vi "CRYOpen Curve Excel .vi"(11 "file path (dialog if empty)":path=path "D:/3_Doc/KTH/test excel/CRY6151 Data Col.csv") -> (0 "Return":bool, 3 "Data":T1[](array[typedef]) {"Z data" items=["dB", "Lin"]; "X data" items=["dB", "Lin"]; "Y data" items=["dB", "Lin"]; "Z dB ref" format="%.1f"; "Z axis" items=["Log", "Lin"]; "X dB ref" format="%.1f"; "X axis" items=["Log", "Lin"]; "Y axis" items=["Log", "Lin"]; "Y dB ref" format="%.1f"; "Curve"."z" format="%.2f"; "Curve"."y" format="%.2f"; "Curve"."x" format="%.2f"})   [LabVIEW 2013]
uses:
  Typedef Control/CRYData Cluster.ctl
  <vilib>/Utility/file.llb/Read From Spreadsheet File (string).vi
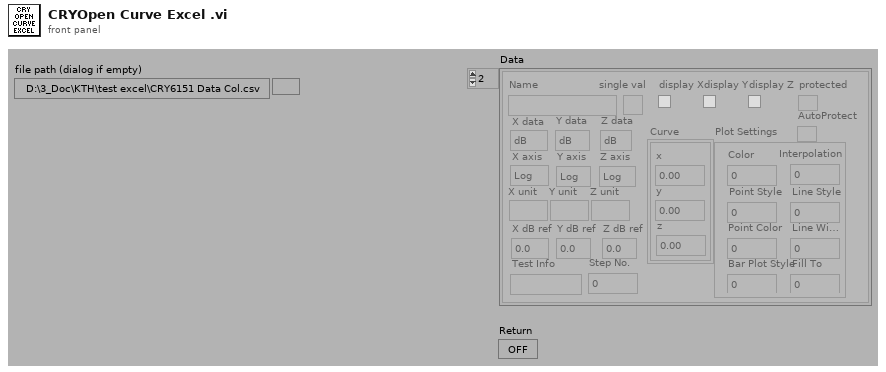
[diagram p1: front panel]
types:
  T1 = typedef "CRYData Cluster.ctl" = cluster{"Name":string, "Curve":cluster{"x":dbl, "y":dbl, "z":dbl}[], "X data":u16, "Y data":u16, "Z data":u16, "X axis":u16, "Y axis":u16, "Z axis":u16, "X unit":string, "Y unit":string, "Z unit":string, "X dB ref":dbl, "Y dB ref":dbl, "Z dB ref":dbl, "single val":bool, "protected":bool, "display X":bool, "display Y":bool, "display Z":bool, "Test Info":string, "Step No.":i32, "Plot Settings":cluster{"Color":u32, "Interpolation":u8, "Point Style":u8, "Line Style":u8, "Point Color":u32, "Line Width":u8, "Bar Plot Style":u8, "Fill To":i16}, "AutoProtect":bool}
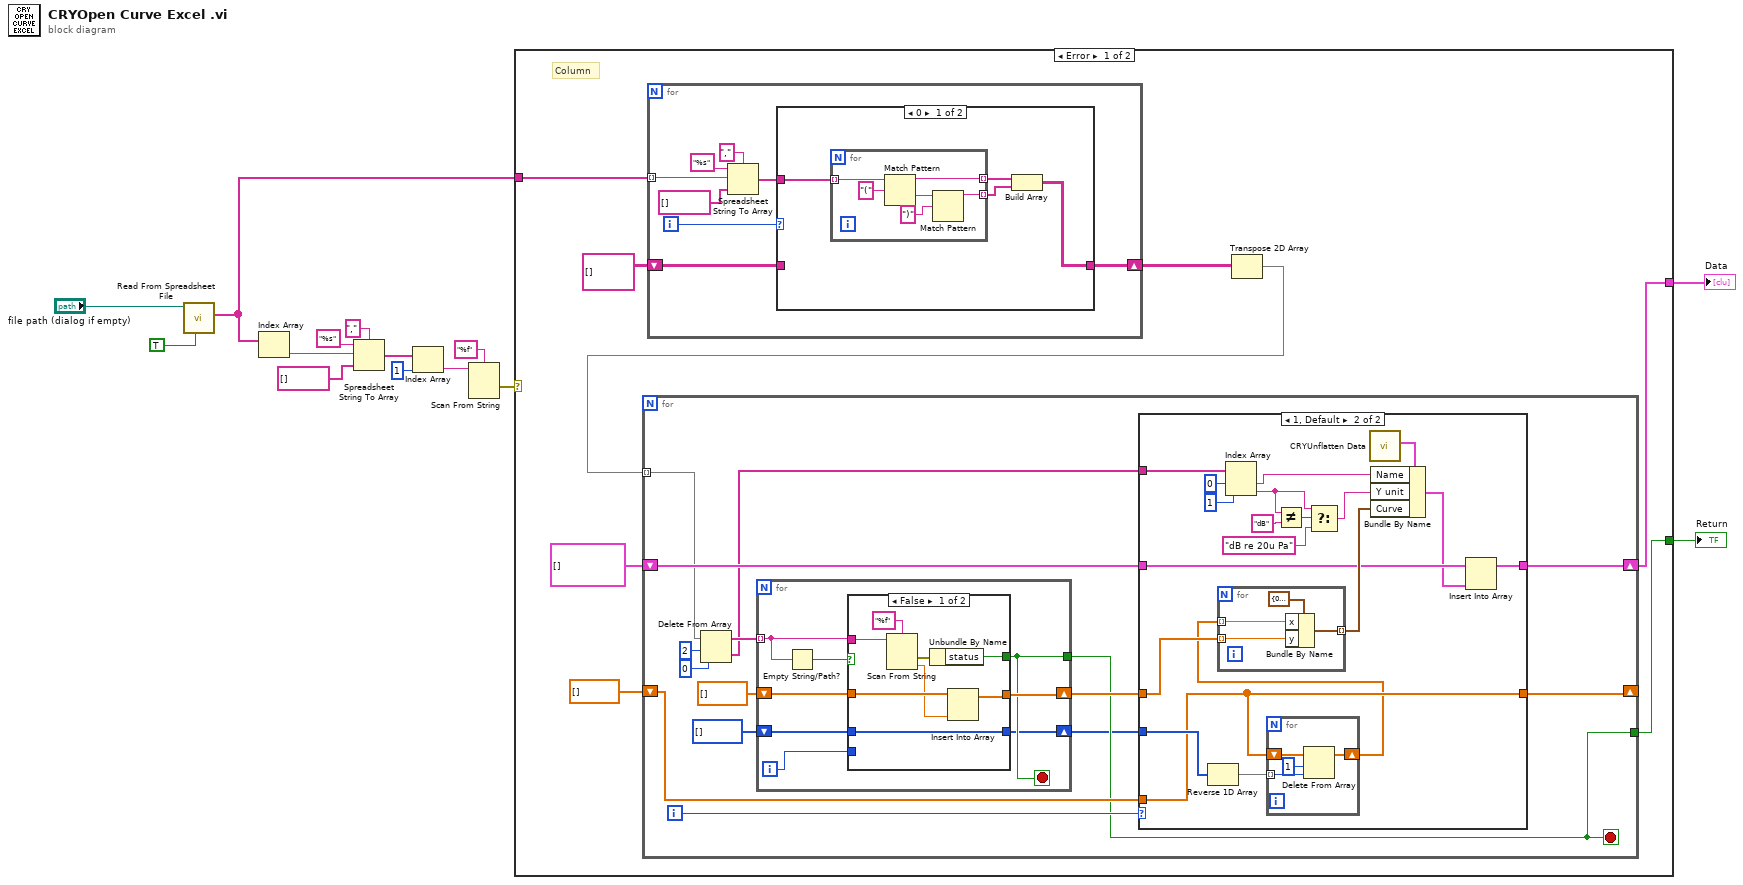
[diagram p0: block diagram]
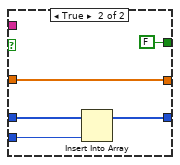
[diagram p3: hidden frame]
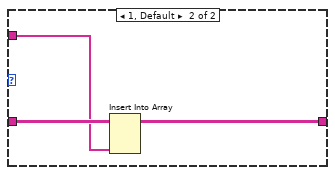
[diagram p4: hidden frame]
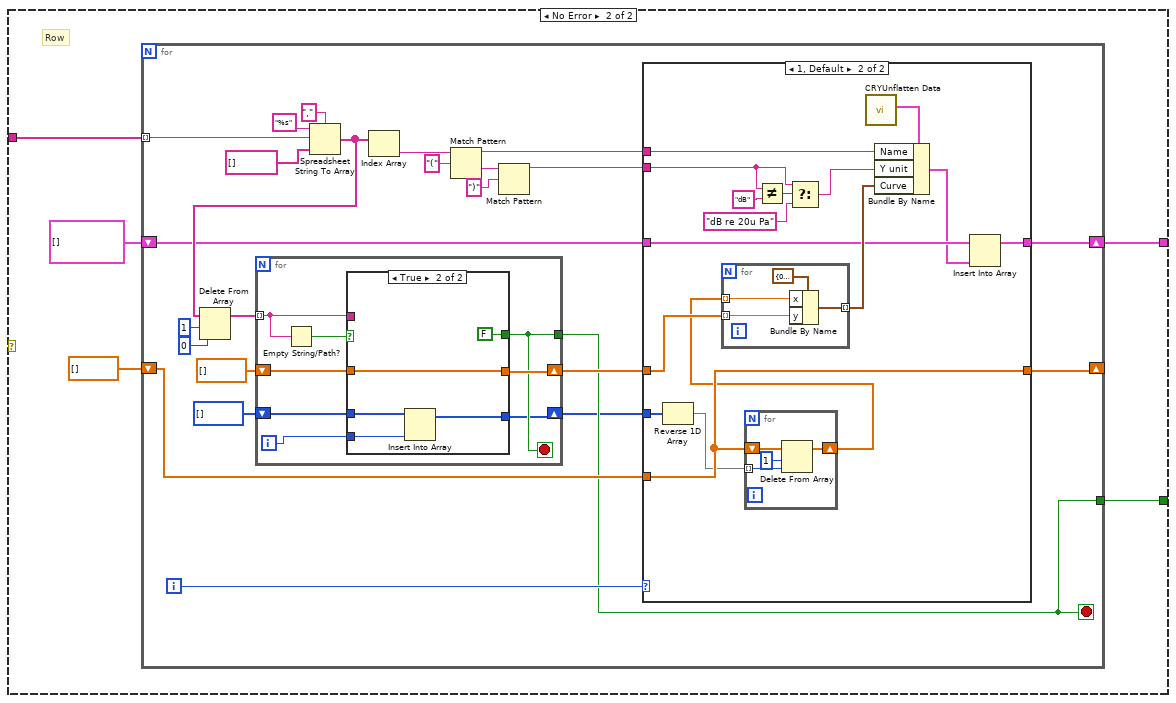
[diagram p5: hidden frame]
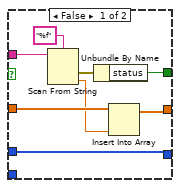
[diagram p7: hidden frame]
diagram:
  n1 = call-poly <vilib>:"Read From Spreadsheet File.vi"("transpose (no:F)"=TRUE, "file path (dialog if empty)"="file path (dialog if empty)") -> ("first row"=w3:string[])  [unwired: 5 in, 4 out]
  n2 = Index Array(array=w3) -> (element=w8:string)  [unwired: 1 in]
  n3 = Spreadsheet String To Array(delimiter (Tab)=",", format string="%s", spreadsheet string=w8, array type (2D Dbl)=string[] []) -> (array=w12:string[])
  n4 = Index Array(array=w12, index=1) -> (element=w5:string)
  n5 = Scan From String(format string="%f", input string=w5) -> (error out=w2:errorcluster)  [unwired: 4 in, 2 out]
  n6 = case shown="Error" w2 {
    tunnel: [w16 w111] -> w4
    tunnel: w3 -> [w22 w110]
    tunnel: [w15 w109] -> w1
    frame Error {
      # "Column"
      n7 = for {
        tunnel: w22 -> [w95] mode=indexing
        shift-right: [w88] -> w20
        shift-left: string[][] [] ("appended array") -> [w89]
        i -> [w90]
        n8 = Spreadsheet String To Array(delimiter (Tab)=",", format string="%s", spreadsheet string=w95, array type (2D Dbl)=string[] []) -> (array=w91:string[])
        n9 = case shown="0" w90 {
          tunnel: w91 -> [w99 w107]
          tunnel: [w97 w106] -> w88
          tunnel: w89 -> [_ w108]
          frame 0 {
            n10 = for {
              tunnel: w99 -> [w100] mode=indexing
              tunnel: [w102] -> w98 mode=indexing
              tunnel: [w101] -> w96 mode=indexing
              n11 = Match Pattern(string=w100, regular expression="(" ("search string/char (-)")) -> (before substring=w102:string, after substring=w105:string)  [unwired: 1 in, 2 out]
              n12 = Match Pattern(string=w105, regular expression=")") -> (before substring=w101:string)  [unwired: 1 in, 3 out]
            }
            n13 = Build Array(w98, w96) -> (w97:string[][])
          }
          frame 1, Default {
            n14 = Insert Into Array(array=w108, new element=w107) -> (w106:string[][])  [unwired: 2 in]
          }
        }
      }
      n15 = Transpose 2D Array(2D array=w20) -> (transposed array=w17:string[][])
      n16 = for {
        tunnel: w17 -> [w27] mode=indexing
        shift-right: [w31] -> _
        shift-left: dbl[] [] -> [w30]
        shift-right: [w28] -> w16
        shift-left: T1[] [] -> [w29]
        tunnel: [w25] -> w15
        i -> [w33]
        stop <- w25 stop-if-true
        n17 = Delete From Array(array=w27, length=2, index=0) -> (deleted portion=w26:string[], array with subset deleted=w35:string[])
        n18 = for {
          tunnel: w35 -> [w74] mode=indexing
          shift-right: [w71] -> w32
          shift-left: dbl[] [] -> [w72]
          tunnel: [w70] -> w25
          shift-right: [w68] -> w23
          shift-left: i32[] [] -> [w69]
          i -> [w67]
          stop <- w70 stop-if-true
          n19 = Empty String/Path?(string/path=w74) -> (empty?=w73:bool)
          n20 = case shown="False" w73 {
            tunnel: w74 -> [w81 _]
            tunnel: w72 -> [w80 w87]
            tunnel: [w79 w87] -> w71
            tunnel: [w76 FALSE ("status")] -> w70
            tunnel: w69 -> [w75 w85]
            tunnel: [w75 w84] -> w68
            tunnel: w67 -> [_ w83]
            frame False {
              n21 = Scan From String(format string="%f", input string=w81) -> (error out=w77:errorcluster, output 1=w78:dbl)  [unwired: 3 in, 2 out]
              n22 = Unbundle By Name(w77) -> ("status"=w76:bool)
              n23 = Insert Into Array(array=w80, new element=w78) -> (w79:dbl[])  [unwired: 1 in]
            }
            frame True {
              n24 = Insert Into Array(array=w85, new element=w83) -> (w84:i32[])  [unwired: 1 in]
            }
          }
        }
        n25 = case shown="1, Default" w33 {
          tunnel: w32 -> [w39 w56]
          tunnel: [w39 w46] -> w31
          tunnel: w30 -> [_ w46]
          tunnel: w29 -> [w38 w55]
          tunnel: [w38 w53] -> w28
          tunnel: w26 -> [_ w52]
          tunnel: w23 -> [_ w47]
          frame 0 {
          }
          frame 1, Default {
            n26 = Reverse 1D Array(array=w47) -> (reversed array=w48:i32[])
            n27 = Index Array(array=w52, index #1=0 ("index"), index #2=1 ("index")) -> (element #1=w49:string, element #2=w42:string)
            n28 = for {
              shift-right: [w59] -> w45
              shift-left: w46 -> [w62]
              tunnel: w48 -> [w61] mode=indexing
              n29 = Delete From Array(array=w62, length=1, index=w61) -> (array with subset deleted=w59:dbl[])  [unwired: 1 out]
            }
            n30 = for {
              tunnel: [w65] -> w57 mode=indexing
              tunnel: w45 -> [w64] mode=indexing
              tunnel: w56 -> [w63] mode=indexing
              n31 = Bundle By Name(cluster=cluster{"x":dbl, "y":dbl, "z":dbl} {"x"=0.0, "y"=0.0, "z"=0.0}, "x"=w64, "y"=w63) -> (w65:cluster{"x":dbl, "y":dbl, "z":dbl})
            }
            n32 = Not Equal?(x=w42, y="dB" ("element")) -> (x != y?=w44:bool)
            n33 = Select(t=w42, s=w44, f="dB re 20u Pa") -> (s? t:f=w40:string)
            n34 = call "CRYUnflatten Data.vi"() -> ("Datum"=w58:T1)  [unwired: 9 in, 2 out]
            n35 = Bundle By Name(cluster=w58, "Name"=w49, "Y unit"=w40, "Curve"=w57) -> (w54:T1)
            n36 = Insert Into Array(array=w55, new element=w54) -> (w53:T1[])  [unwired: 1 in]
          }
        }
      }
    }
    frame No Error {
      # "Row"
      n37 = for {
        tunnel: w110 -> [w137] mode=indexing
        shift-right: [w120] -> _
        shift-left: dbl[] [] -> [w119]
        shift-right: [w117] -> w111
        shift-left: T1[] [] -> [w118]
        tunnel: [w116] -> w109
        i -> [w122]
        stop <- w116 stop-if-true
        n38 = Spreadsheet String To Array(delimiter (Tab)=",", format string="%s", spreadsheet string=w137, array type (2D Dbl)=string[] []) -> (array=w125:string[])
        n39 = Delete From Array(array=w125, length=1, index=0) -> (array with subset deleted=w124:string[])  [unwired: 1 out]
        n40 = for {
          tunnel: w124 -> [w171] mode=indexing
          shift-right: [w168] -> w121
          shift-left: dbl[] [] -> [w169]
          tunnel: [w167] -> w116
          shift-right: [w165] -> w114
          shift-left: i32[] [] -> [w166]
          i -> [w164]
          stop <- w167 stop-if-true
          n41 = Empty String/Path?(string/path=w171) -> (empty?=w170:bool)
          n42 = case shown="True" w170 {
            tunnel: w171 -> [w178 _]
            tunnel: w169 -> [w177 w184]
            tunnel: [w176 w184] -> w168
            tunnel: [w173 FALSE ("status")] -> w167
            tunnel: w166 -> [w172 w182]
            tunnel: [w172 w181] -> w165
            tunnel: w164 -> [_ w180]
            frame False {
              n43 = Scan From String(format string="%f", input string=w178) -> (error out=w174:errorcluster, output 1=w175:dbl)  [unwired: 3 in, 2 out]
              n44 = Unbundle By Name(w174) -> ("status"=w173:bool)
              n45 = Insert Into Array(array=w177, new element=w175) -> (w176:dbl[])  [unwired: 1 in]
            }
            frame True {
              n46 = Insert Into Array(array=w182, new element=w180) -> (w181:i32[])  [unwired: 1 in]
            }
          }
        }
        n47 = Index Array(array=w125) -> (element=w136:string)  [unwired: 1 in]
        n48 = Match Pattern(string=w136, regular expression="(" ("search string/char (-)")) -> (before substring=w135:string, after substring=w134:string)  [unwired: 1 in, 2 out]
        n49 = Match Pattern(string=w134, regular expression=")") -> (before substring=w131:string)  [unwired: 1 in, 3 out]
        n50 = case shown="1, Default" w122 {
          tunnel: w135 -> [_ w154]
          tunnel: w131 -> [_ w141]
          tunnel: w121 -> [w139 w152]
          tunnel: [w139 w148] -> w120
          tunnel: w119 -> [_ w148]
          tunnel: w118 -> [w138 w151]
          tunnel: [w138 w149] -> w117
          tunnel: w114 -> [_ w147]
          frame 0 {
          }
          frame 1, Default {
            n51 = Reverse 1D Array(array=w147) -> (reversed array=w146:i32[])
            n52 = for {
              shift-right: [w156] -> w145
              shift-left: w148 -> [w159]
              tunnel: w146 -> [w158] mode=indexing
              n53 = Delete From Array(array=w159, length=1, index=w158) -> (array with subset deleted=w156:dbl[])  [unwired: 1 out]
            }
            n54 = for {
              tunnel: [w162] -> w153 mode=indexing
              tunnel: w145 -> [w161] mode=indexing
              tunnel: w152 -> [w160] mode=indexing
              n55 = Bundle By Name(cluster=cluster{"x":dbl, "y":dbl, "z":dbl} {"x"=0.0, "y"=0.0, "z"=0.0}, "x"=w161, "y"=w160) -> (w162:cluster{"x":dbl, "y":dbl, "z":dbl})
            }
            n56 = Not Equal?(x=w141, y="dB" ("element")) -> (x != y?=w144:bool)
            n57 = Select(t=w141, s=w144, f="dB re 20u Pa") -> (s? t:f=w140:string)
            n58 = call "CRYUnflatten Data.vi"() -> ("Datum"=w155:T1)  [unwired: 9 in, 2 out]
            n59 = Bundle By Name(cluster=w155, "Name"=w154, "Y unit"=w140, "Curve"=w153) -> (w150:T1)
            n60 = Insert Into Array(array=w151, new element=w150) -> (w149:T1[])  [unwired: 1 in]
          }
        }
      }
    }
  }
  "Data" <- w4
  "Return" <- w1
